vi "TEST Array Indexing.vi"() -> ()   [LabVIEW 2013, in "Carya Config.lvclass"]
doc: "Copyright 2018, Carya Automatisering, Wiebe Walstra."
uses:
  Carya Config.lvclass
  CConfig Variant Accessor/CConfig Variant Accessor.lvclass
panel:
  out "String 2":string
  out "section_key":dbl
  out "String":string="[section 1]\nkey 1=2\nkey 2=2\nkey 3=2\nkey 4=2\n\nkey 7=2\r\nkey 8=2\r\n[section 2]\ngdfgsd=32\r\n[section 3]\r\nkey 12=2"
  # "Should return the values that are set as defaults."
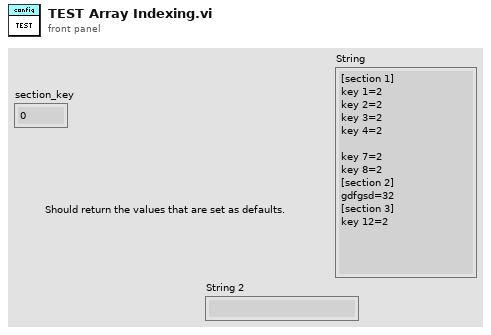
[diagram p1: front panel]
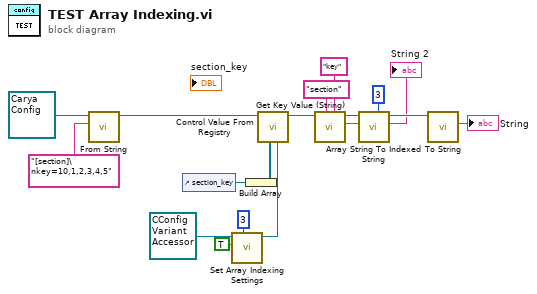
[diagram p0: block diagram]
diagram:
  n1 = call-dynamic "From String.vi"("String"="[section]\nkey=10,1,2,3,4,5", "Carya Config in"=refnum<class "Carya Config.lvclass"> refnum) -> ("Carya Config out"=w16:refnum<class "Carya Config.lvclass">)  [unwired: 7 in, 2 out]
  n2 = control-ref of="section_key"() -> (w13:refnum<vi>)
  n3 = call "Set Array Indexing Settings.vi"("Index [-1]"=3, "Array indexing [F]"=TRUE, "CConfig Variant Accessor in"=refnum<class "CConfig Variant Accessor.lvclass"> refnum) -> ("CConfig Variant Accessor out"=w11:refnum<class "CConfig Variant Accessor.lvclass">)  [unwired: 7 in, 1 out]
  n4 = Build Array(w13) -> (w12:refnum<vi>[])
  n5 = call "Control Value From Registry.vi"("Registry Variant Accessor (optional)"=w11, "Controls"=w12, "Registry Object in"=w16) -> ("Registry Object out"=w14:refnum<class "Carya Config.lvclass">)  [unwired: 6 in, 2 out]
  n6 = call "Get Key Value (String).vi"("Key name"="key" ("Section name"), "Section name"="section", "Carya Config in"=w14) -> ("Value"=w5:string, "Carya Config out"=w7:refnum<class "Carya Config.lvclass">)  [unwired: 5 in, 2 out]
  n7 = call-dynamic "Array String To Indexed String.vi"("Index [0]"=3, "String (RAW)"=w5, "Registry Object"=w7) -> ("String"=→"String 2":string, "Registry Object"=w6:refnum<class "Carya Config.lvclass">)  [unwired: 6 in, 1 out]
  n8 = call-dynamic "To String.vi"("Carya Config in"=w6) -> ("String"=→"String":string)  [unwired: 8 in, 2 out]
